vi "rest invent.vi"(8 "error in (no error)":errorcluster, 9 "Numeric":u16, 10 "Prods":string[][](array[string]), 11 "Nestle Actor in":refnum<class "Nestle Actor.lvclass">) -> (0 "error out":errorcluster, 3 "Nestle Actor out":refnum<class "Nestle Actor.lvclass">)   [LabVIEW 2020, in "Nestle Actor.lvlib" / "Nestle Actor.lvclass"]
uses:
  Nestle Actor.lvclass
  C:/Program Files (x86)/National Instruments/LabVIEW 2020/vi.lib/ActorFramework/Actor/Actor.lvclass
  Nestle Actor.lvclass/Nestle Actor.ctl
  <vilib>/ActorFramework/Actor/Actor.lvclass/Actor.ctl
  UI Actor Messages/Compras Msg/Compras Msg.lvclass/Compras Msg.ctl
  <vilib>/ActorFramework/Message Enqueuer/Message Enqueuer.lvclass/Message Enqueuer.ctl
  <vilib>/ActorFramework/Message Enqueuer/Enqueue.vi
  UI Actor Messages/Compras Msg/Compras Msg.lvclass
  C:/Program Files (x86)/National Instruments/LabVIEW 2020/vi.lib/ActorFramework/Message/Message.lvclass
  <vilib>/ActorFramework/Message Priority Queue/Priority Enqueue.vi
  <vilib>/ActorFramework/Actor/Actor.lvclass
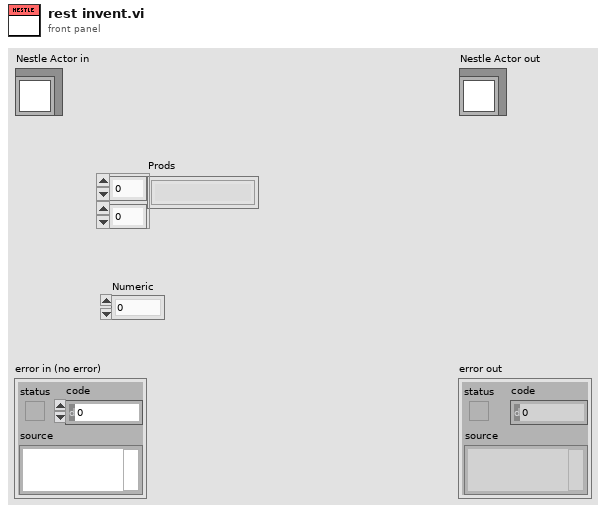
[diagram p1: front panel]
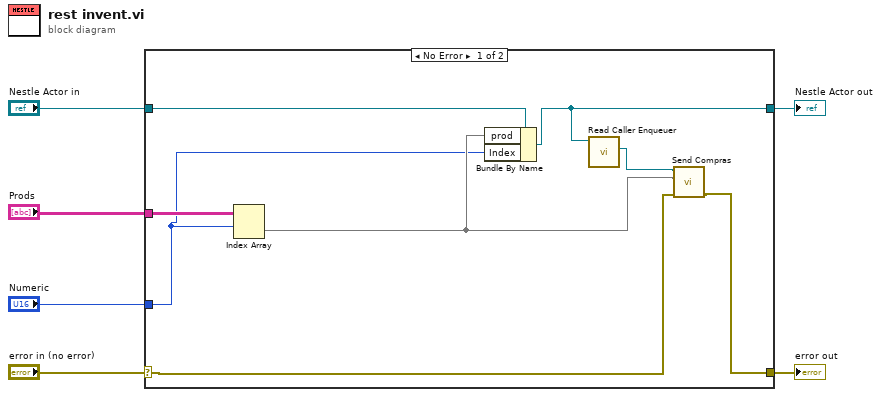
[diagram p0: block diagram]
diagram:
  n1 = case shown="No Error" "error in (no error)" {
    selector: "error in (no error)" -> [w11 w16]
    tunnel: [w10 w16] -> w5
    tunnel: [w8 w15] -> w3
    tunnel: "Nestle Actor in" -> [w12 w15]
    tunnel: "Prods" -> [w13 _]
    tunnel: "Numeric" -> [w7 _]
    frame No Error {
      n2 = Index Array "Index Array"(array=w13, index (row)=w7) -> (element=w9:string[])  [unwired: 1 in]
      n3 = Bundle By Name(cluster=w12, "prod"=w9, "Index"=w7) -> (w8:refnum<class "Nestle Actor.lvclass">)
      n4 = call <vilib>:"Read Caller Enqueuer.vi"("Actor"=w8) -> ("Caller Enqueuer"=w14:refnum<class "Message Enqueuer.lvclass">)  [unwired: 10 in]
      n5 = call "Send Compras.vi"("error in (no error)"=w11, "product"=w9, "Message Enqueuer"=w14) -> ("error out"=w10:errorcluster)  [unwired: 7 in, 1 out]
    }
    frame Error {
    }
  }
  "error out" <- w5
  "Nestle Actor out" <- w3
